vi "setWristAngle.vi"() -> ()   [LabVIEW 2015]
uses:
  ARM angles.vi
panel:
  in  "wr":dbl
  out "old wr":i32
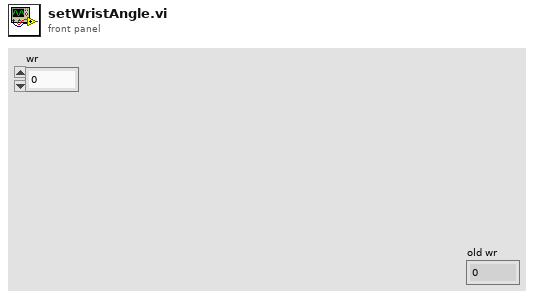
[diagram p1: front panel]
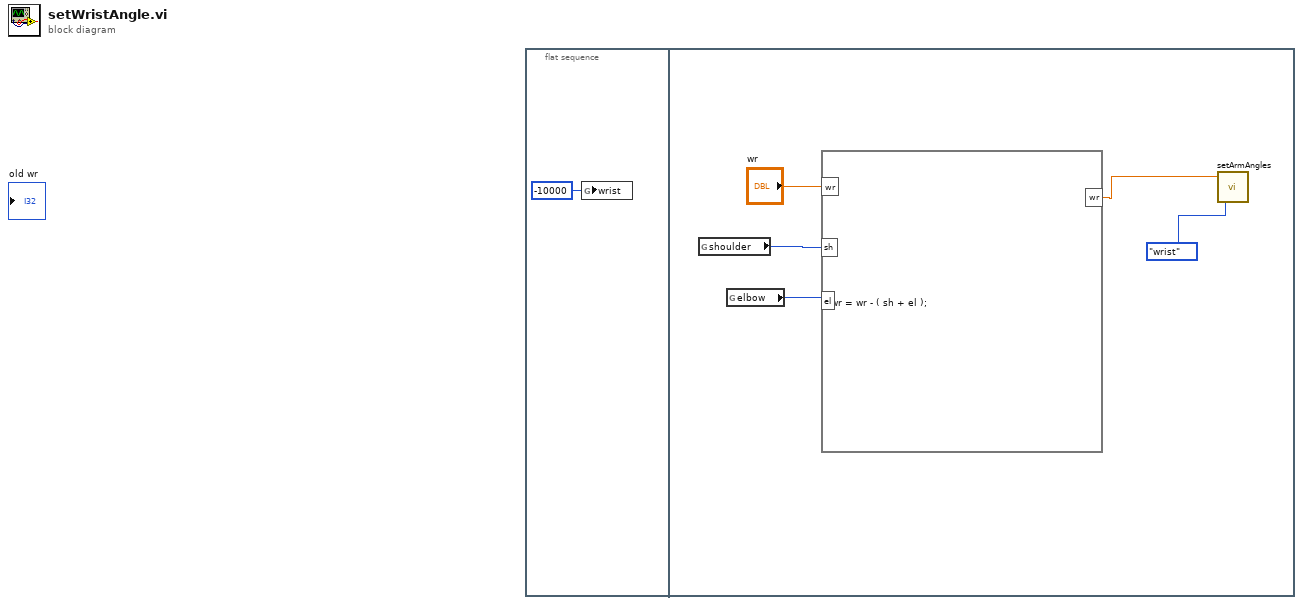
[diagram p0: block diagram]
diagram:
  n1 = flat-sequence {
    frame #0 {
      n2 = global write "ARM angles.vi" "wrist"(-10000 ("wrist")) -> ()
    }
    frame #1 {
      n3 = global read "ARM angles.vi" "shoulder"() -> (w4:i32)
      n4 = global read "ARM angles.vi" "elbow"() -> (w5:i32)
      n5 = formula code="wr = wr - ( sh + el );"("wr"="wr", "sh"=w4, "el"=w5) -> ("wr"=w2:dbl)
      n6 = call "setArmAngles.vi"("Enum"=enum16{"shoulder", "elbow", "wrist"}."wrist", "angle"=w2) -> ()  [unwired: 2 in]
    }
  }
